vi "ReadVNA.vi"(7 "Data Type":T2, 8 "error in (no error)":errorcluster, 10 "VNACluster In":T3={"Value"=0.0, "GUI Data Cluster"={"S11"=FALSE, "S21"=FALSE, "S12"=FALSE, "S22"=FALSE, "S11Meas"=enum."Log-magnitude (dB)", "S21Meas"=enum."Log-magnitude (dB)", "S12Meas"=enum."Log-magnitude (dB)", "S22Meas"=enum."Log-magnitude (dB)"}, "Timing"={"Last Operation"=0.0, "Stop @ T/B"=FALSE, "Last Temp"=0.0, "Last Mag"=0.0, "Ramp Param"={"End T (K)"=0.0, "Delta T (K)"=0.0, "End B (T)"=0.0, "Delta B (T)"=0.0}, "LastOp?"=FALSE}, "Measurements"=[], "Hardware"={"VNA TCP Con"=refnum, "VNA TCP Port"=5025, "Global T VAR"="", "Global B VAR"=""}, "Operation"={"Operation Mode"=enum."Logging", "Log Folder"=path "", "Measure Mode"=enum."Deltat"}}, 11 "Param":enum16{"S11", "S21", "S12", "S22"}(ring)) -> (0 "error out":errorcluster, 1 "Array":dbl[](array[numeric]), 2 "VNACluster Out":T3={"Value"=0.0, "GUI Data Cluster"={"S11"=FALSE, "S21"=FALSE, "S12"=FALSE, "S22"=FALSE, "S11Meas"=enum."Log-magnitude (dB)", "S21Meas"=enum."Log-magnitude (dB)", "S12Meas"=enum."Log-magnitude (dB)", "S22Meas"=enum."Log-magnitude (dB)"}, "Timing"={"Last Operation"=0.0, "Stop @ T/B"=FALSE, "Last Temp"=0.0, "Last Mag"=0.0, "Ramp Param"={"End T (K)"=0.0, "Delta T (K)"=0.0, "End B (T)"=0.0, "Delta B (T)"=0.0}, "LastOp?"=FALSE}, "Measurements"=[], "Hardware"={"VNA TCP Con"=refnum, "VNA TCP Port"=5025, "Global T VAR"="", "Global B VAR"=""}, "Operation"={"Operation Mode"=enum."Logging", "Log Folder"=path "", "Measure Mode"=enum."Deltat"}}, 4 "SweepParam":T1)   [LabVIEW 2021]
uses:
  Sources/Data_Cluster.ctl
  Sources/Measurement_Cluster.ctl
  Sources/Mode_Enum.ctl
  VNA_DataType.ctl
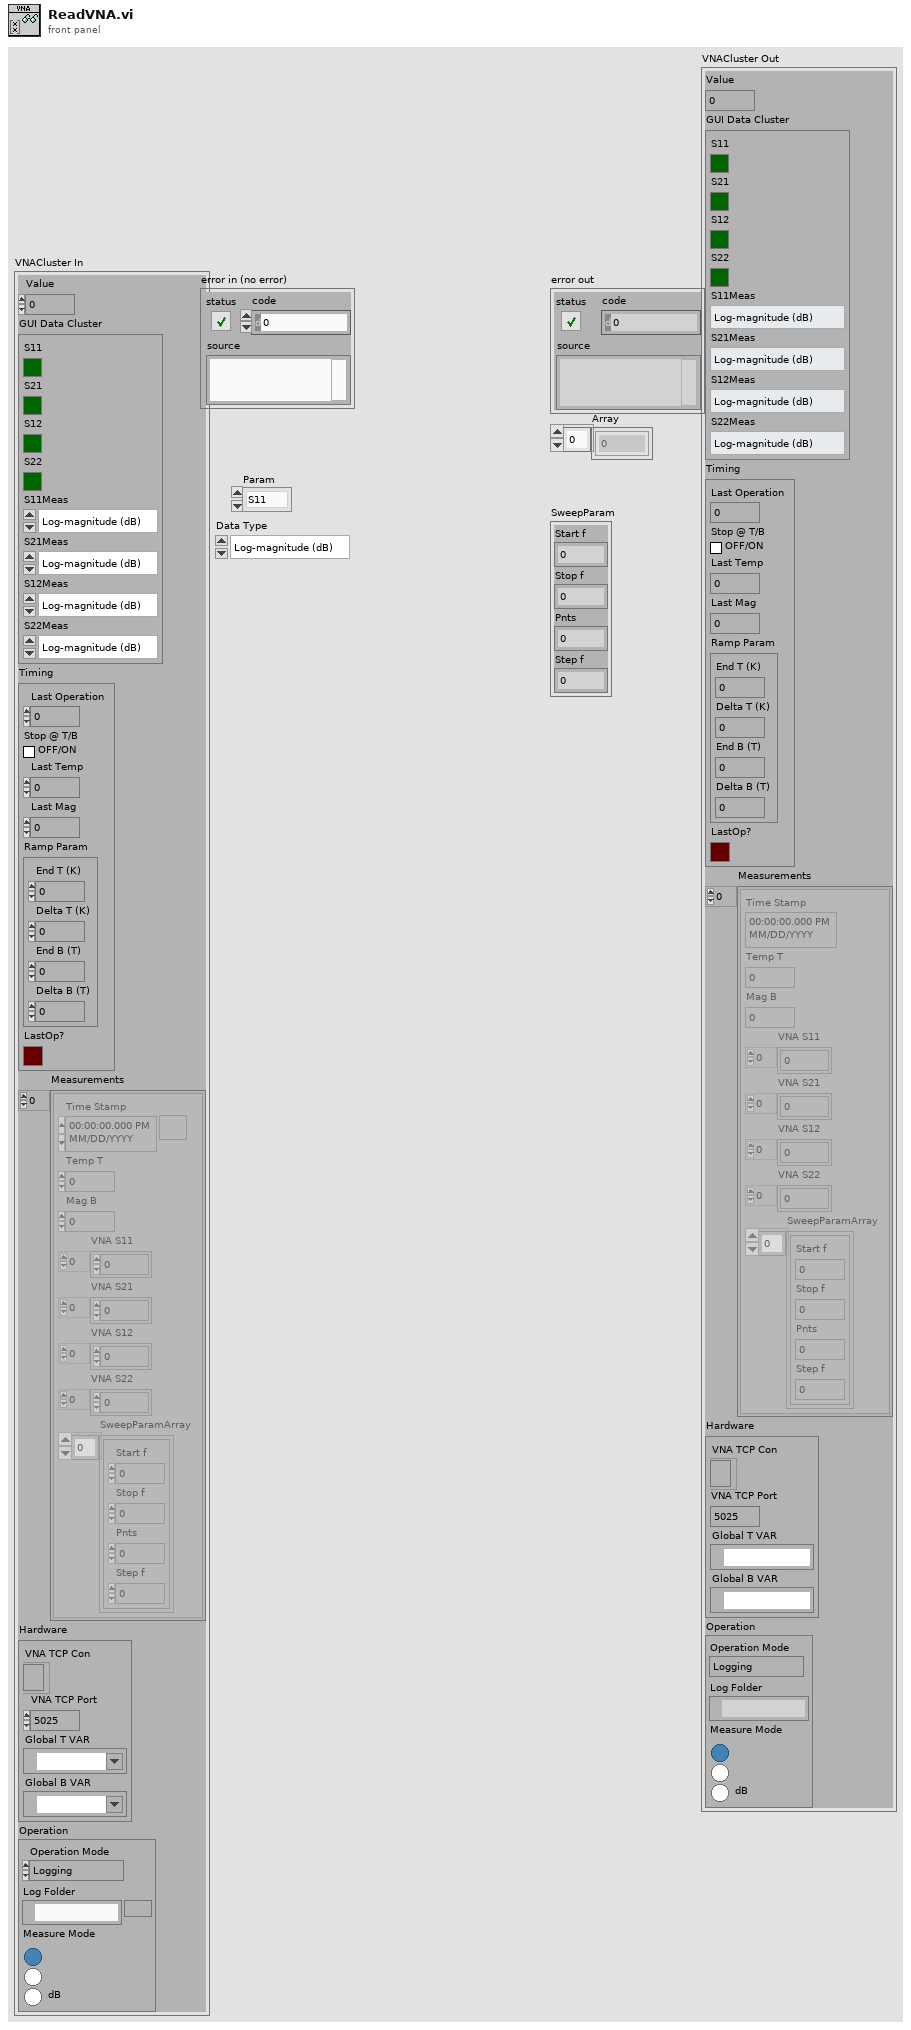
[diagram p1: front panel]
types:
  T1 = cluster{"Start f":dbl, "Stop f":dbl, "Pnts":i32, "Step f":dbl}
  T2 = typedef "VNA_DataType.ctl" = enum16{"Log-magnitude (dB)", "Linear magnitude", "Phase (deg)", "Time Domain", "Real", "Imaginary", "Group Delay", "Polarlinear"}
  T3 = typedef "Data_Cluster.ctl" = cluster{"Value":dbl, "GUI Data Cluster":cluster{"S11":bool, "S21":bool, "S12":bool, "S22":bool, "S11Meas":enum16{"Log-magnitude (dB)", "Linear magnitude", "Phase (deg)", "Time Domain", "Real", "Imaginary", "Group Delay", "Polarlinear"}, "S21Meas":enum16{"Log-magnitude (dB)", "Linear magnitude", "Phase (deg)", "Time Domain", "Real", "Imaginary", "Group Delay", "Polarlinear"}, "S12Meas":enum16{"Log-magnitude (dB)", "Linear magnitude", "Phase (deg)", "Time Domain", "Real", "Imaginary", "Group Delay", "Polarlinear"}, "S22Meas":enum16{"Log-magnitude (dB)", "Linear magnitude", "Phase (deg)", "Time Domain", "Real", "Imaginary", "Group Delay", "Polarlinear"}}, "Timing":cluster{"Last Operation":dbl, "Stop @ T/B":bool, "Last Temp":dbl, "Last Mag":dbl, "Ramp Param":cluster{"End T (K)":dbl, "Delta T (K)":dbl, "End B (T)":dbl, "Delta B (T)":dbl}, "LastOp?":bool}, "Measurements":T4[], "Hardware":cluster{"VNA TCP Con":refnum<k5>, "VNA TCP Port":i32, "Global T VAR":refnum<k21>, "Global B VAR":refnum<k21>}, "Operation":cluster{"Operation Mode":T5, "Log Folder":path, "Measure Mode":enum32{"Deltat", "DeltaT", "dB"}}}
  T4 = typedef "Measurement_Cluster.ctl" = cluster{"Time Stamp":timestamp, "Temp T":dbl, "Mag B":dbl, "VNA S11":dbl[], "VNA S21":dbl[], "VNA S12":dbl[], "VNA S22":dbl[], "SweepParamArray":cluster{"Start f":dbl, "Stop f":dbl, "Pnts":i32, "Step f":dbl}[]}
  T5 = typedef "Mode_Enum.ctl" = enum16{"Logging", "Idle-Off", "Idle"}
  T6 = enum16{"Standard", "Buffered", "CRLF", "Immediate"}
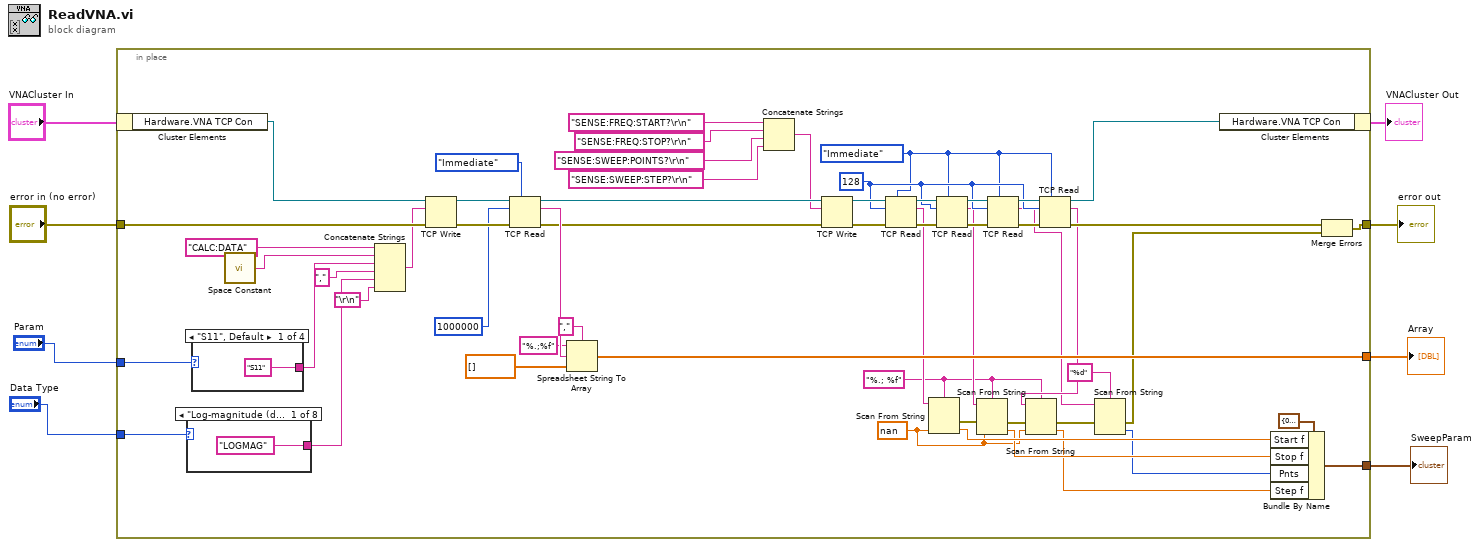
[diagram p0: block diagram]
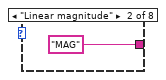
[diagram p2: hidden frame]
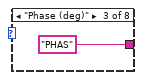
[diagram p3: hidden frame]
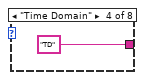
[diagram p4: hidden frame]
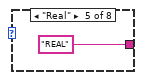
[diagram p5: hidden frame]
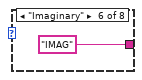
[diagram p6: hidden frame]
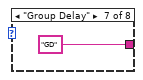
[diagram p7: hidden frame]
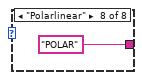
[diagram p8: hidden frame]
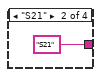
[diagram p9: hidden frame]
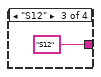
[diagram p10: hidden frame]
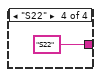
[diagram p11: hidden frame]
diagram:
  n1 = in-place {
    in-place-border: "error in (no error)" -> [w65]
    in-place-border: [w25] -> w5
    in-place-border: "Param" -> [w57]
    in-place-border: "Data Type" -> [w55]
    in-place-border: [w46] -> w2
    in-place-border: [w22] -> w1
    w16 = nan
    w14 = "%.; %f" ("format string")
    w29 = T6."Immediate" ("mode (standard)")
    w30 = 128 ("bytes to read")
    n2 = in-place-cluster #1("VNACluster In") -> ("Hardware.VNA TCP Con"=w64:refnum<k5>)
    n3 = case shown="\"Log-magnitude (dB)\", Default" w55 {
      tunnel: ["LOGMAG" "MAG" "PHAS" "TD" "REAL" "IMAG" "GD" "POLAR"] -> w53
      frame "Log-magnitude (dB)", Default {
      }
      frame "Linear magnitude" {
      }
      frame "Phase (deg)" {
      }
      frame "Time Domain" {
      }
      frame "Real" {
      }
      frame "Imaginary" {
      }
      frame "Group Delay" {
      }
      frame "Polarlinear" {
      }
    }
    n4 = case shown="\"S11\", Default" w57 {
      tunnel: ["S11" "S21" "S12" "S22"] -> w56
      frame "S11", Default {
      }
      frame "S21" {
      }
      frame "S12" {
      }
      frame "S22" {
      }
    }
    n5 = call <vilib>:"Space Constant.vi"() -> ("String"=w58:string)
    n6 = Concatenate Strings("CALC:DATA" ("string"), w58, w56, ",", w53, "\r\n") -> (w51:string)
    n7 = TCP Write(connection ID=w64, data in=w51, error in (no error)=w65) -> (connection ID out=w62:refnum<k5>, error out=w63:errorcluster)  [unwired: 1 in, 1 out]
    n8 = TCP Read(connection ID=w62, bytes to read=1000000, error in (no error)=w63, 7:T6."Immediate" ("mode (standard)")) -> (connection ID out=w44:refnum<k5>, data out=w50:string, error out=w45:errorcluster)  [unwired: 1 in]
    n9 = Spreadsheet String To Array(delimiter (Tab)=",", format string="%.;%f", spreadsheet string=w50, array type (2D Dbl)=dbl[] []) -> (array=w46:dbl[])
    n10 = Concatenate Strings("SENSE:FREQ:START?\r\n" ("data in"), "SENSE:FREQ:STOP?\r\n" ("data in"), "SENSE:SWEEP:POINTS?\r\n" ("data in"), "SENSE:SWEEP:STEP?\r\n" ("data in")) -> (w39:string)
    n11 = TCP Write(connection ID=w44, data in=w39, error in (no error)=w45) -> (connection ID out=w37:refnum<k5>, error out=w38:errorcluster)  [unwired: 1 in, 1 out]
    n12 = TCP Read(connection ID=w37, bytes to read=w30, error in (no error)=w38, 7:w29) -> (connection ID out=w36:refnum<k5>, data out=w27:string, error out=w35:errorcluster)  [unwired: 1 in]
    n13 = Scan From String(format string=w14, input string=w27, default 1=w16) -> (error out=w20:errorcluster, output 1=w23:dbl)  [unwired: 2 in, 2 out]
    n14 = TCP Read(connection ID=w36, bytes to read=w30, error in (no error)=w35, 7:w29) -> (connection ID out=w32:refnum<k5>, data out=w21:string, error out=w34:errorcluster)  [unwired: 1 in]
    n15 = Scan From String(format string=w14, input string=w21, error in=w20, default 1=w16) -> (error out=w18:errorcluster, output 1=w19:dbl)  [unwired: 1 in, 2 out]
    n16 = TCP Read(connection ID=w32, bytes to read=w30, error in (no error)=w34, 7:w29) -> (connection ID out=w31:refnum<k5>, data out=w13:string, error out=w33:errorcluster)  [unwired: 1 in]
    n17 = TCP Read(connection ID=w31, bytes to read=w30, error in (no error)=w33, 7:w29) -> (connection ID out=w28:refnum<k5>, data out=w17:string, error out=w26:errorcluster)  [unwired: 1 in]
    n18 = Scan From String(format string=w14, input string=w17, error in=w18, default 1=w16) -> (error out=w11:errorcluster, output 1=w15:dbl)  [unwired: 1 in, 2 out]
    n19 = Scan From String(format string="%d", input string=w13, error in=w11) -> (error out=w9:errorcluster, output 1=w10:i32)  [unwired: 2 in, 2 out]
    n20 = in-place-cluster #1("Hardware.VNA TCP Con"=w28) -> (→"VNACluster Out":T3)
    n21 = Bundle By Name(cluster=T1 {"Start f"=0.0, "Stop f"=0.0, "Pnts"=0, "Step f"=0.0} ("SweepParam"), "Start f"=w23, "Stop f"=w19, "Pnts"=w10, "Step f"=w15) -> (w22:T1)
    n22 = Merge Errors(w26, w9) -> (w25:errorcluster)
  }
  "error out" <- w5
  "Array" <- w2
  "SweepParam" <- w1
